vi "getChildEvents.vi"(8 "error in (no error)":errorcluster, 11 "CommandEvents in":refnum<class "CommandEvents.lvclass">) -> (0 "error out":errorcluster, 2 "Events":T1, 3 "CommandEvents out":refnum<class "CommandEvents.lvclass">)   [LabVIEW 2009, in "Tools.lvlib" / "Interpreters.lvlib" / "CommandEvents.lvclass"]
uses:
  CommandEvents.lvclass
  CommandEvents.lvclass/CommandEvents.ctl
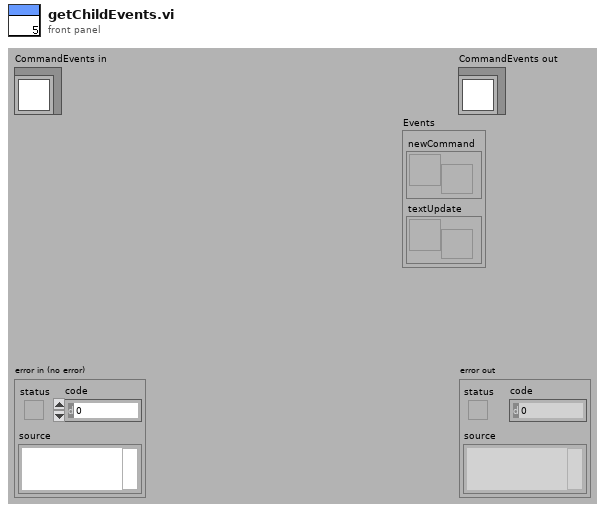
[diagram p1: front panel]
types:
  T1 = cluster{"newCommand":refnum<user-event>, "textUpdate":refnum<user-event>}
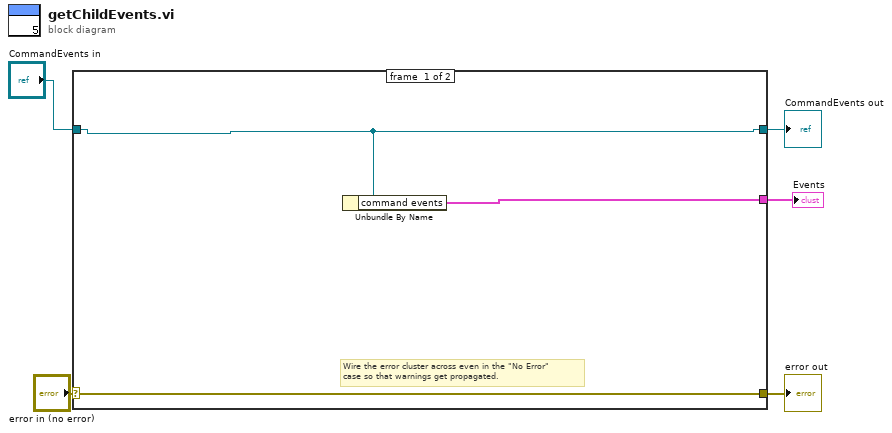
[diagram p0: block diagram]
diagram:
  n1 = case shown="No Error" "error in (no error)" {
    selector: "error in (no error)" -> [w8 w10]
    tunnel: [w8 w10] -> w4
    tunnel: [w6 w9] -> w2
    tunnel: "CommandEvents in" -> [w6 w9]
    tunnel: [w7 _] -> w1
    frame #0 {
      # "Wire the error cluster across even in the \"No Error\"\ncase so that warnings get propagated."
      n2 = Unbundle By Name(w6) -> ("command events"=w7:T1)
    }
    frame #1 {
    }
  }
  "error out" <- w4
  "CommandEvents out" <- w2
  "Events" <- w1
